vi "Set70dbAtten.vi"(2 "error in (no error)":errorcluster, 3 "Attenuation (dB)":i32=70 min=0 max=120 step=10 format="%_3g") -> (0 "error out":errorcluster)   [LabVIEW 2009]
doc: "Opens channel for specified ID"
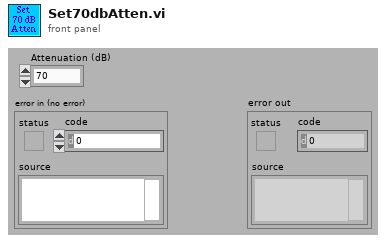
[diagram p1: front panel]
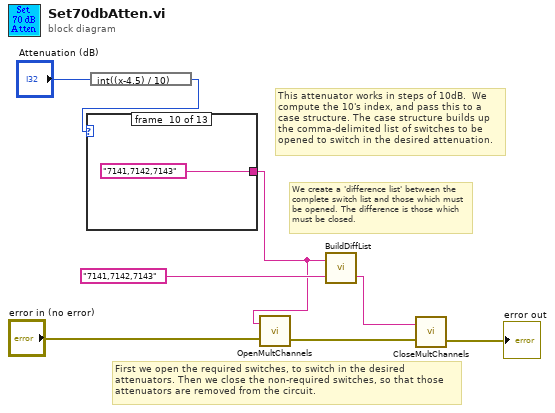
[diagram p0: block diagram]
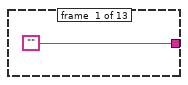
[diagram p2: hidden frame]
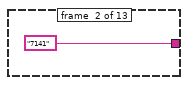
[diagram p3: hidden frame]
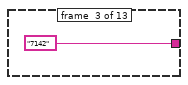
[diagram p4: hidden frame]
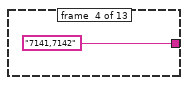
[diagram p5: hidden frame]
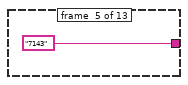
[diagram p6: hidden frame]
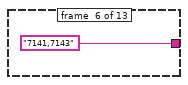
[diagram p7: hidden frame]
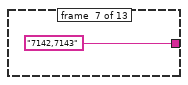
[diagram p8: hidden frame]
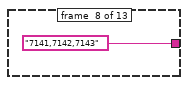
[diagram p9: hidden frame]
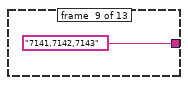
[diagram p10: hidden frame]
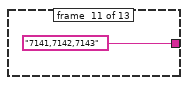
[diagram p11: hidden frame]
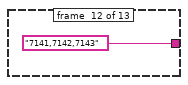
[diagram p12: hidden frame]
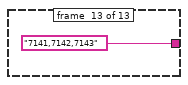
[diagram p13: hidden frame]
diagram:
  # "First we open the required switches, to switch in the desired attenuators. Then we close the non-required switches, so that those attenuators are removed from the circuit."
  # "We create a 'difference list' between the complete switch list and those which must be opened. The difference is those which must be closed."
  # "This attenuator works in steps of 10dB.  We compute the 10's index, and pass this to a case structure. The case structure builds up the comma-delimited list of switches to be opened to switch in the desired attenuation."
  n1 = expression code="int((x-4.5) / 10)"("Attenuation (dB)") -> (w7:i32)
  n2 = case shown="12" w7 {
    tunnel: ["" "7141" "7142" "7141,7142" "7143" "7141,7143" "7142,7143" "7141,7142,7143" "7141,7142,7143" "7141,7142,7143" "7141,7142,7143" "7141,7142,7143" "7141,7142,7143"] -> w1
    frame #0 {
    }
    frame #1 {
    }
    frame #2 {
    }
    frame #3 {
    }
    frame #4 {
    }
    frame #5 {
    }
    frame #6 {
    }
    frame #7 {
    }
    frame #8 {
    }
    frame #9 {
    }
    frame #10 {
    }
    frame #11 {
    }
    frame #12 {
    }
  }
  n3 = call "OpenMultChannels.vi"("error in (no error)"="error in (no error)", "Channels to be opened"=w1) -> ("error out"=w4:errorcluster)  [unwired: 1 in]
  n4 = call "BuildDiffList.vi"("Reference list"="7141,7142,7143", "Input list"=w1) -> ("Difference list"=w2:string)  [unwired: 1 in]
  n5 = call "CloseMultChannels.vi"("error in (no error)"=w4, "Channels to be closed"=w2) -> ("error out"=→"error out":errorcluster)  [unwired: 1 in]
